vi "Parse Ramp To Zero Fault.vi"(11 "Ramp To Zero Fault":u8 format="%02x") -> (3 "Ramp To Zero":T1 {"Ramp To Zero Fault" format="%02x"})   [LabVIEW 2019]
uses:
  Ramp To Zero Display.ctl
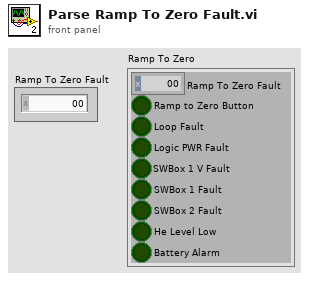
[diagram p1: front panel]
types:
  T1 = typedef "Ramp To Zero Display.ctl" = cluster{"Ramp To Zero Fault":u8, "Ramp to Zero Button":bool, "Loop Fault":bool, "Logic PWR Fault":bool, "SWBox 1 V Fault":bool, "SWBox 1 Fault":bool, "SWBox 2 Fault":bool, "He Level Low":bool, "Battery Alarm":bool}
  T2 = cluster{"Ramp To Zero Fault":u8, bool, bool, bool, bool, bool, bool, bool, bool}
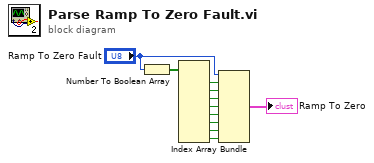
[diagram p0: block diagram]
diagram:
  n1 = Number To Boolean Array(number="Ramp To Zero Fault") -> (Boolean array=w10:bool[])
  n2 = Index Array(array=w10) -> (element #1=w8:bool, element #2=w7:bool, element #3=w6:bool, element #4=w5:bool, element #5=w4:bool, element #6=w3:bool, element #7=w2:bool, element #8=w1:bool)  [unwired: 8 in]
  n3 = Bundle("Ramp To Zero Fault"="Ramp To Zero Fault", w8, w7, w6, w5, w4, w3, w2, w1) -> (→"Ramp To Zero":T2)  [unwired: 1 in]
